vi "GlobalClicksHeight_raw.vi"() -> ()   [LabVIEW 2019]
panel:
  in  "Frame properties (m)":cluster{cluster{dbl, dbl}, cluster{dbl, dbl}}
  in  "Position (nm)":cluster{"X":dbl, "Z":dbl, "Y":dbl}
  in  "Safe Tip?":bool
  in  "Starting Height (nm)":dbl
  out "Setpoint (A)":dbl=100.0
  out "Current (pA)":dbl
  in  "Found Surface?":bool
  out "Surface Location (nm)":dbl
  in  "Starting Height?":bool
  in  "Clicks and Height":bool
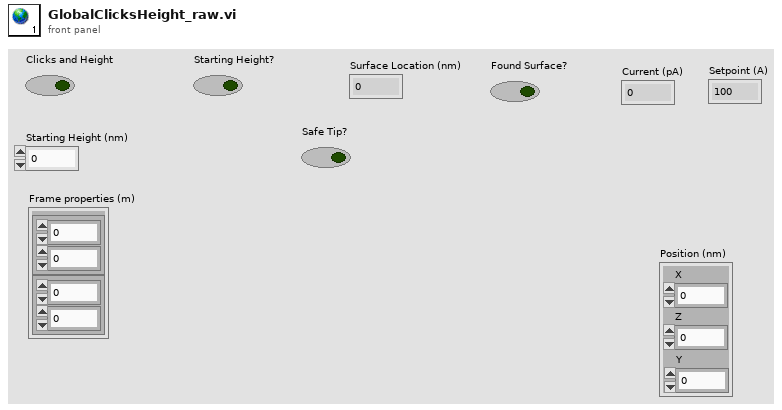
[diagram p1: front panel]
diagram:
